vi "GenerateFilepath.vi"(8 "error in (no error)":errorcluster, 10 "Base path":path, 11 "Experiment in":refnum<class "Experiment.lvclass">) -> (0 "error out":errorcluster, 2 "File":path, 3 "Experiment out":refnum<class "Experiment.lvclass">)   [LabVIEW 2014, in "Experiment.lvclass"]
uses:
  Experiment.lvclass
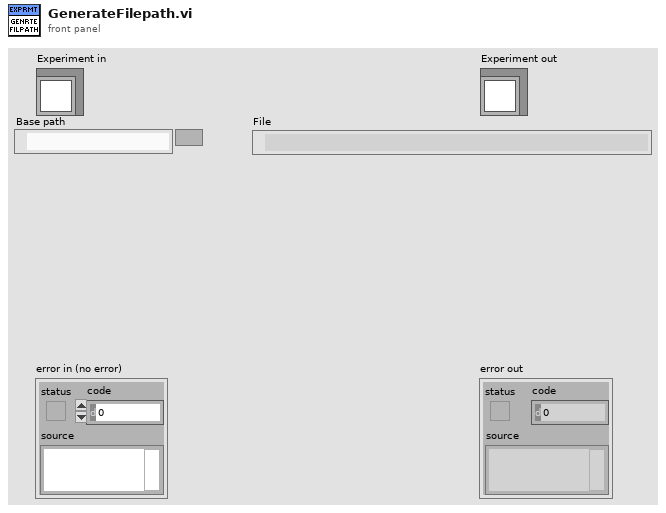
[diagram p1: front panel]
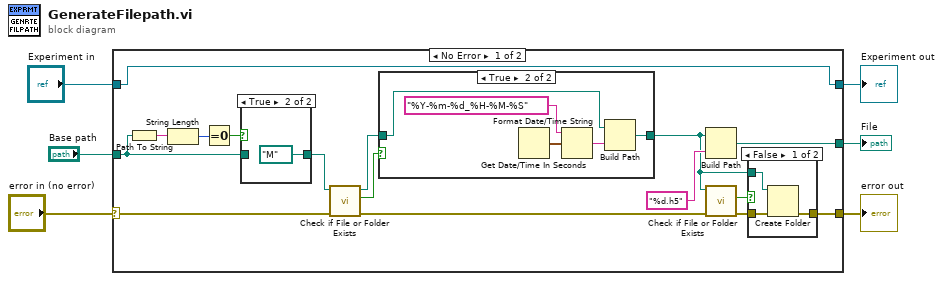
[diagram p0: block diagram]
diagram:
  n1 = case shown="No Error" "error in (no error)" {
    selector: "error in (no error)" -> [w10 w37]
    tunnel: [w9 w37] -> w5
    tunnel: [w7 w36] -> w3
    tunnel: "Experiment in" -> [w7 w36]
    tunnel: "Base path" -> [w12 w35]
    tunnel: [w11 w35] -> w1
    frame No Error {
      n2 = Path To String(path=w12) -> (string=w16:string)
      n3 = String Length(string=w16) -> (length=w15:i32)
      n4 = Equal To 0?(x=w15) -> (x = 0?=w14:bool)
      n5 = case shown="True" w14 {
        tunnel: w12 -> [w23 _]
        tunnel: [w23 path "M:/" ("Base path")] -> w13
        frame False {
        }
        frame True {
        }
      }
      n6 = call <vilib>:"Check if File or Folder Exists.vi"("error in (no error)"=w10, "path"=w13) -> ("error out"=w8:errorcluster, "file or folder exists?"=w17:bool, "dup path"=w18:path)  [unwired: 7 in]
      n7 = case shown="True" w17 {
        tunnel: w18 -> [w25 w28]
        tunnel: [w25 w27] -> w19
        frame False {
        }
        frame True {
          n8 = Get Date/Time In Seconds() -> (seconds since 1Jan1904=w29:timestamp)
          n9 = Format Date/Time String(time format string (%c)="%Y-%m-%d_%H-%M-%S", seconds (now)=w29) -> (date/time string=w30:string)  [unwired: 1 out]
          n10 = Build Path(base path=w28, name or relative path=w30) -> (appended path=w27:path)
        }
      }
      n11 = Build Path(base path=w19, name or relative path="%d.h5" ("string")) -> (appended path=w11:path)
      n12 = call <vilib>:"Check if File or Folder Exists.vi"("error in (no error)"=w8, "path"=w19) -> ("error out"=w21:errorcluster, "file or folder exists?"=w20:bool)  [unwired: 7 in, 1 out]
      n13 = case shown="False" w20 {
        tunnel: w19 -> [w33 _]
        tunnel: w21 -> [w32 w34]
        tunnel: [w31 w34] -> w9
        frame False {
          n14 = Create Folder(path (use dialog)=w33, error in=w32) -> (error out=w31:errorcluster)  [unwired: 1 in, 2 out]
        }
        frame True {
        }
      }
    }
    frame Error {
    }
  }
  "error out" <- w5
  "Experiment out" <- w3
  "File" <- w1
